vi "AppendLog.vi"(1 "error in":errorcluster, 2 "text to write":string, 3 "file path (use dialog)":path) -> (0 "error out":errorcluster)   [LabVIEW 2014]
doc: "Stateless logging of text to disk via appending"
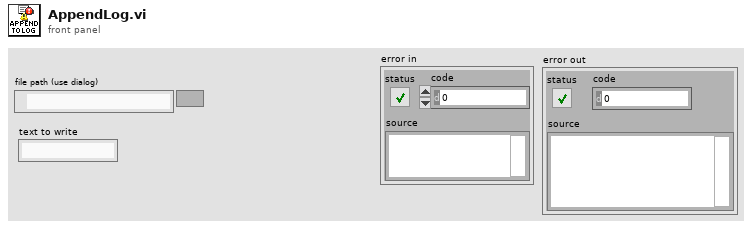
[diagram p1: front panel]
types:
  T1 = enum16{"open", "replace", "create", "open or create", "replace or create", "replace or create with confirmation"}
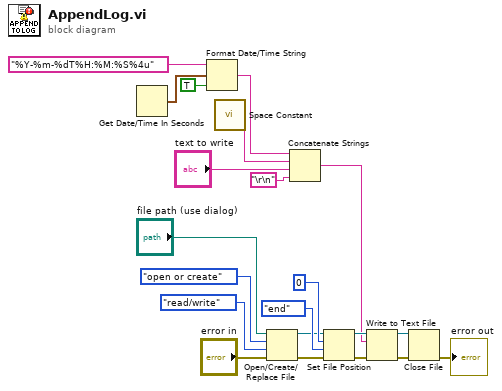
[diagram p0: block diagram]
diagram:
  n1 = Get Date/Time In Seconds() -> (seconds since 1Jan1904=w9:timestamp)
  n2 = Format Date/Time String(time format string (%c)="%Y-%m-%dT%H:%M:%S%4u", seconds (now)=w9, UTC format=TRUE) -> (date/time string=w7:string)
  n3 = call <vilib>:"Space Constant.vi"() -> ("String"=w5:string)
  n4 = Open/Create/Replace File(file path (use dialog)="file path (use dialog)", error in="error in", operation (0:open)=T1."open or create", access (0:read/write)=enum16{"read/write", "read-only", "write-only"}."read/write") -> (refnum out=w13:refnum<file>, error out=w16:errorcluster)  [unwired: 2 in, 1 out]
  n5 = Concatenate Strings(w7, w5, "text to write", "\r\n") -> (w2:string)
  n6 = Set File Position(offset (in bytes) (0)=i64 0, refnum=w13, from (0:start)=enum16{"start", "end", "current"}."end", error in=w16) -> (refnum out=w18:refnum<file>, error out=w17:errorcluster)
  n7 = Write to Text File(file (use dialog)=w18, text=w2, error in=w17) -> (refnum out=w20:refnum<file>, error out=w21:errorcluster)  [unwired: 1 in, 1 out]
  n8 = Close File(refnum=w20, error in=w21) -> (error out=→"error out":errorcluster)  [unwired: 1 out]
